vi "explore_events.vi"() -> ()   [LabVIEW 2023]
panel:
  out "error out 2":errorcluster
  out "return type":i32
  out "decimal integer string":string
  out "cnt":i32
  out "*(type *) &x":i32
  out "error out":errorcluster
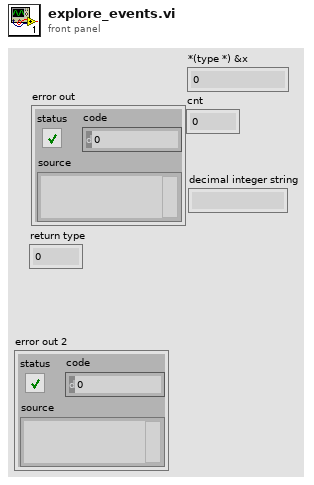
[diagram p1: front panel]
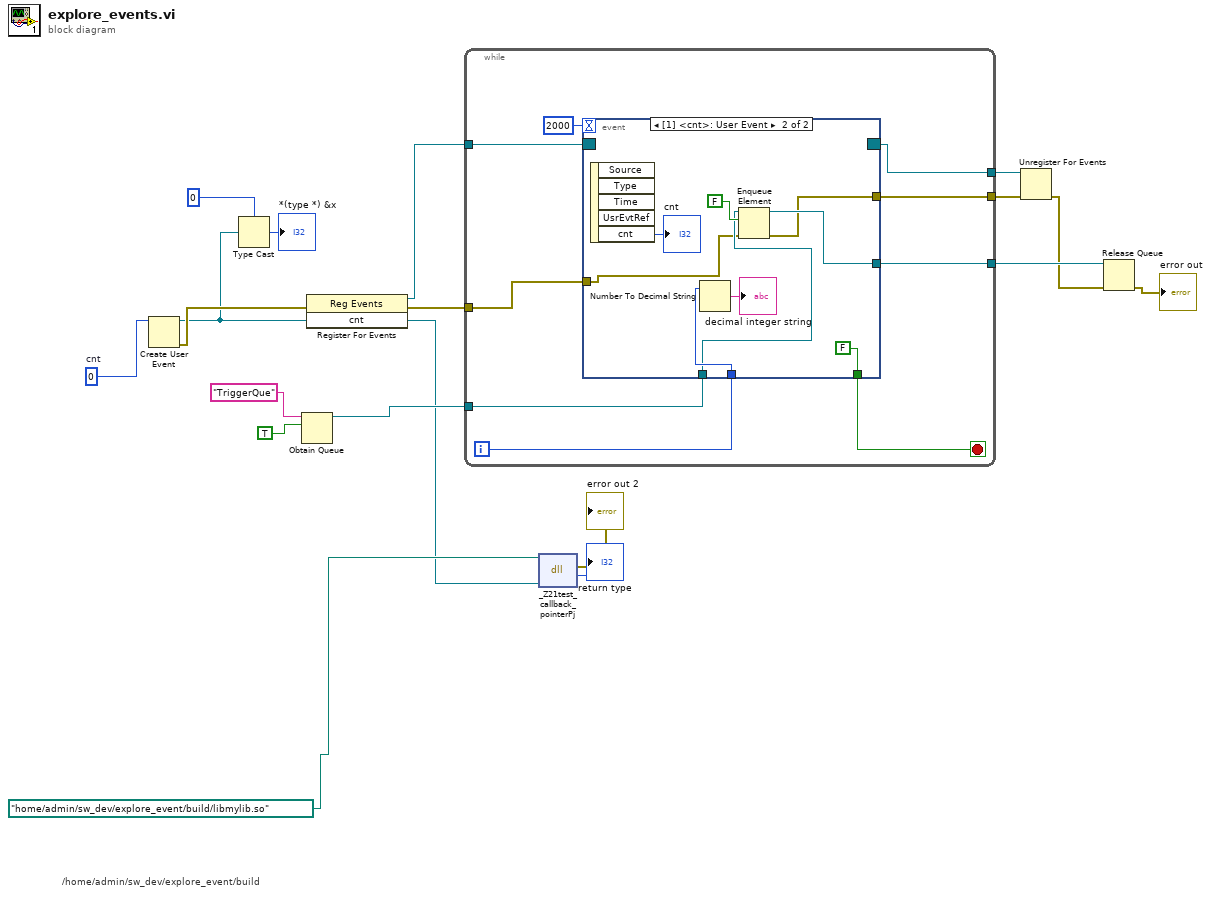
[diagram p0: block diagram]
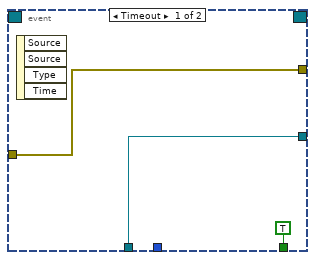
[diagram p2: hidden frame]
diagram:
  w16 = 0  # cnt
  # "/home/admin/sw_dev/explore_event/build"
  n1 = Create User Event(user event datatype=w16) -> (user event=w3:refnum<user-event>, error out=w5:errorcluster)  [unwired: 1 in]
  n2 = Type Cast(type=0, x=w3) -> (*(type *) &x=→"*(type *) &x":i32)
  n3 = Obtain Queue(name (unnamed)="TriggerQue", element data type=TRUE) -> (queue out=w12:refnum<queue>)  [unwired: 3 in, 2 out]
  n4 = register-events(error in=w5, w3) -> (reference out=w18:refnum<event-registration>, error out=w11:errorcluster)  [unwired: 1 in]
  n5 = while {
    tunnel: w18 -> [w27]
    tunnel: [w26] -> w17
    tunnel: w12 -> [w24]
    tunnel: w11 -> [w23]
    tunnel: [w21] -> w10
    tunnel: [w20] -> w8
    i -> [w25]
    stop <- w19 stop-if-true
    n6 = event shown="[1] <cnt>: User Event" {
      selector: w27 -> [_ _]
      dyn-events: [_ _] -> w26
      timeout: 2000 -> [_ _]
      tunnel: w25 -> [_ w38]
      tunnel: w24 -> [w30 w35]
      tunnel: w23 -> [w29 w33]
      tunnel: [w30 w34] -> w21
      tunnel: [w29 w32] -> w20
      tunnel: [TRUE FALSE] -> w19
      event Timeout {
        n7 = event-data() -> ()  [unwired: 1 in, 4 out]
      }
      event User Event {
        n8 = event-data() -> ("cnt"=→"cnt":i32)  [unwired: 1 in, 4 out]
        n9 = Number To Decimal String(number=w38) -> (decimal integer string=→"decimal integer string":string)  [unwired: 1 in]
        n10 = Enqueue Element(queue=w35, element=FALSE, error in (no error)=w33) -> (queue out=w34:refnum<queue>, error out=w32:errorcluster)  [unwired: 1 in, 1 out]
      }
    }
  }
  n11 = dll-call lib="libmylib.so" fn="_Z21test_callback_pointerPj"(path in=path "/home/admin/sw_dev/explore_event/build/libmylib.so", "ref"=w3) -> (error out=→"error out 2":errorcluster, "return type"=→"return type":i32)  [unwired: 3 in, 1 out]
  n12 = Unregister For Events(event registration refnum=w17, error in=w8) -> (error out=w7:errorcluster)
  n13 = Release Queue(queue=w10, error in (no error)=w7) -> (error out=→"error out":errorcluster)  [unwired: 1 in, 2 out]
